vi "Set Dynamic Resolution Parameters [DRE].vi"(7 "Micropulse # In":i32, 8 "error in (no error)":errorcluster, 9 "DRE Hysteresis Delay":u8, 10 "DRE Gain":T1, 11 "Test No.":u32) -> (0 "error out":errorcluster, 5 "Micropulse # Out":i32)   [LabVIEW 2026, in "MicroPulse_Driver.lvlib"]
uses:
  MicroPulse_Driver.lvlib
  Data/Datatypes/MP - DRE gain.ctl
  Private/MP-Registry Action-Enum.ctl
  <instrlib>/Micropulse/Micropulse.lvlib
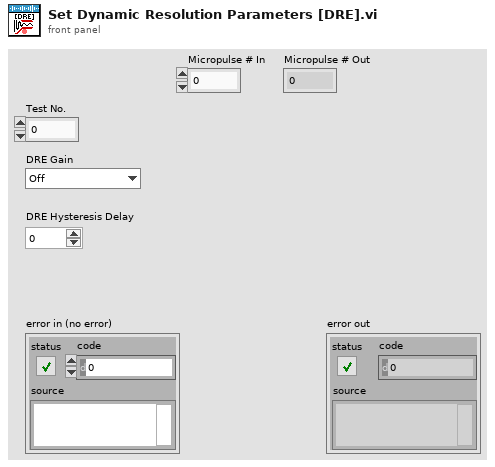
[diagram p1: front panel]
types:
  T1 = typedef "Micropulse.lvlib/MP - DRE gain.ctl" = enum16{"Off", "30dB", "36dB", "42dB", "48dB"}
  T2 = typedef "MicroPulse_Driver.lvlib/MP-Registry Action-Enum.ctl" = enum16{"Read", "Add Test", "Add Command", "Add Gate Command", "Add Encoder Command", "Clear Command  List", "Set Registry", "Set System Details", "Set DOF", "Set Velocity", "Disable Asynch Reads", "Enable Asynch Reads", "Add Connection", "Disconnect", "Shutdown"}
  T3 = typedef "Micropulse.lvlib/TCP config.ctl" = cluster{"Connection ID":refnum<k5>, "IP address":string, "host port":u16, "OC timeout":i32, "Read timeout":i32, "Write timeout":i32}
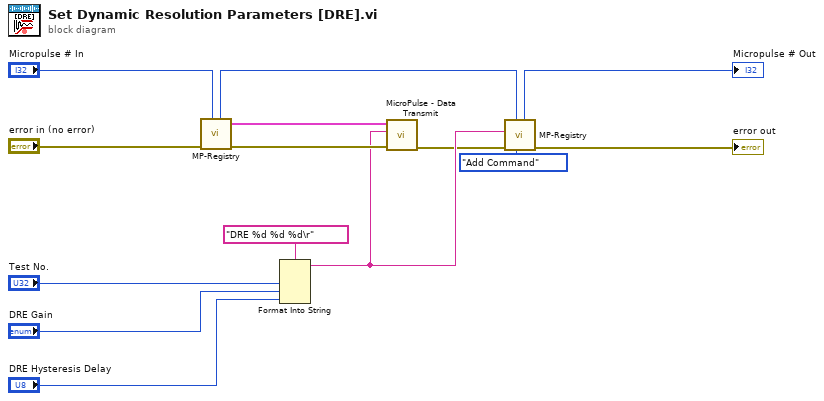
[diagram p0: block diagram]
diagram:
  n1 = call "MP-Registry.vi"("Micropulse # In"="Micropulse # In", "error in (no error)"="error in (no error)") -> ("error out"=w12:errorcluster, "TCP config"=w11:T3, "Micropulse # Out"=w7:i32)  [unwired: 6 in, 1 out]
  n2 = Format Into String(format string="DRE %d %d %d\r", "Test No.", "DRE Gain", "DRE Hysteresis Delay") -> (resulting string=w10:string)  [unwired: 2 in, 1 out]
  n3 = call "MicroPulse - Data Transmit.vi"("error in (no error)"=w12, "data"=w10, "TCP config"=w11) -> ("error out"=w8:errorcluster)  [unwired: 6 in, 2 out]
  n4 = call "MP-Registry.vi"("Action"=MP-Registry_Action-Enum."Add Command", "Micropulse # In"=w7, "error in (no error)"=w8, "Data in"=w10) -> ("error out"=→"error out":errorcluster, "Micropulse # Out"=→"Micropulse # Out":i32)  [unwired: 4 in, 2 out]
